vi "Check If Multiple LV Instances Allowed.vi"(8 "error in":errorcluster) -> (0 "error out":errorcluster, 3 "Multiple LV Instances allowed?":bool)   [LabVIEW 2015, in "CLI.lvclass"]
doc: "This VI determines whether this application instance could receive command line arguments.\nIn Development System it checks labview.ini file for \"allowmultipleinstances\" flag.\nIn Run Time Engine, outputs True, even if given exe is not allowed to run in multiple instances."
uses:
  CLI.lvclass
  <vilib>/Utility/config.llb/NI_LVConfig.lvlib
  <vilib>/Utility/config.llb/Read Key (Boolean).vi
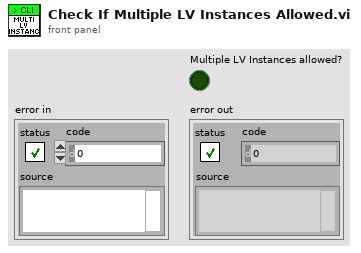
[diagram p1: front panel]
types:
  T1 = typedef "NI_LVConfig.lvlib/Config Data RefNum.ctl" = refnum<k1>
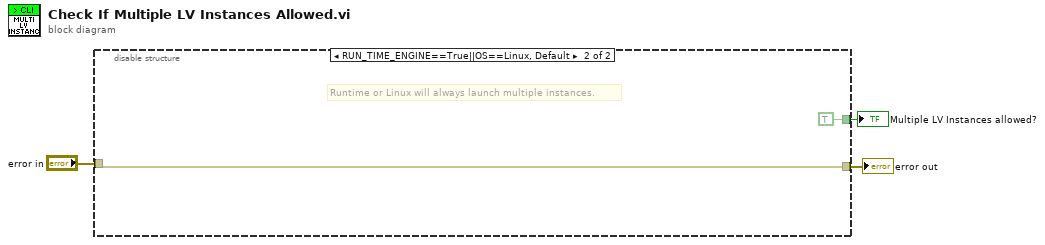
[diagram p0: block diagram]
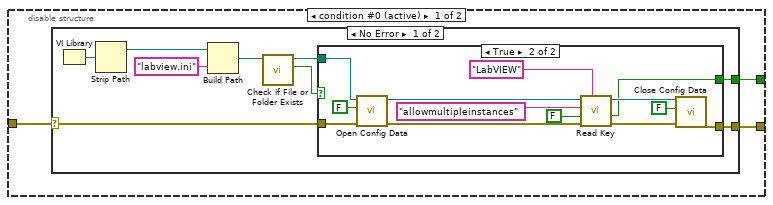
[diagram p2: hidden frame]
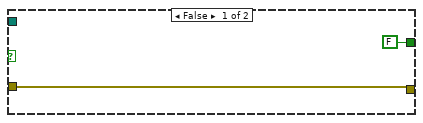
[diagram p3: hidden frame]
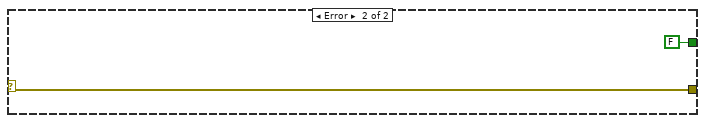
[diagram p4: hidden frame]
diagram:
  n1 = disable-structure shown="RUN_TIME_ENGINE==True||OS==Linux, Default" {
    disable-tunnel: [w6 TRUE ("value")] -> w3
    disable-tunnel: [w5 w34] -> w2
    disable-tunnel: "error in" -> [w4 w34]
    frame condition #0 (active) {
      n2 = case shown="No Error" w4 {
        selector: w4 -> [w8 w31]
        tunnel: [w12 FALSE ("value")] -> w6
        tunnel: [w11 w31] -> w5
        frame No Error {
          n3 = VI Library() -> (path=w15:path)
          n4 = Strip Path(path=w15) -> (stripped path=w14:path)  [unwired: 1 out]
          n5 = Build Path(base path=w14, name or relative path="labview.ini") -> (appended path=w10:path)
          n6 = call <vilib>:"Check if File or Folder Exists.vi"("path"=w10) -> ("file or folder exists?"=w7:bool, "dup path"=w9:path)  [unwired: 8 in, 1 out]
          n7 = case shown="True" w7 {
            tunnel: [FALSE ("value") w21] -> w12
            tunnel: w8 -> [w17 w20]
            tunnel: [w17 w19] -> w11
            tunnel: w9 -> [_ w18]
            frame False {
            }
            frame True {
              n8 = call <vilib>:"Open Config Data.vi"("error in (no error)"=w20, "create file if necessary (T)"=FALSE, "configuration file path"=w18) -> ("error out"=w29:errorcluster, "refnum"=w28:T1)  [unwired: 6 in, 1 out]
              n9 = call-poly <vilib>:"Read Key.vi"("section"="LabVIEW", "error in (no error)"=w29, "default value"=FALSE, "key"="allowmultipleinstances", "refnum"=w28) -> ("error out"=w24:errorcluster, "value"=w21:bool, "refnum out"=w23:T1)  [unwired: 3 in, 1 out]
              n10 = call <vilib>:"Close Config Data.vi"("error in (no error)"=w24, "write file if changed (T)"=FALSE, "refnum"=w23) -> ("error out"=w19:errorcluster)  [unwired: 7 in, 1 out]
            }
          }
        }
        frame Error {
        }
      }
    }
    frame condition #1 {
      # "Runtime or Linux will always launch multiple instances."
    }
  }
  "Multiple LV Instances allowed?" <- w3
  "error out" <- w2
